vi "Log_Errors_20190313.vi"(7 "LoopName":string, 10 "error in":errorcluster) -> (2 "error out":errorcluster)   [LabVIEW 2021]
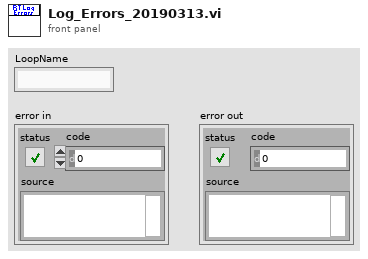
[diagram p1: front panel]
types:
  T1 = enum16{"open", "replace", "create", "open or create", "replace or create", "replace or create with confirmation"}
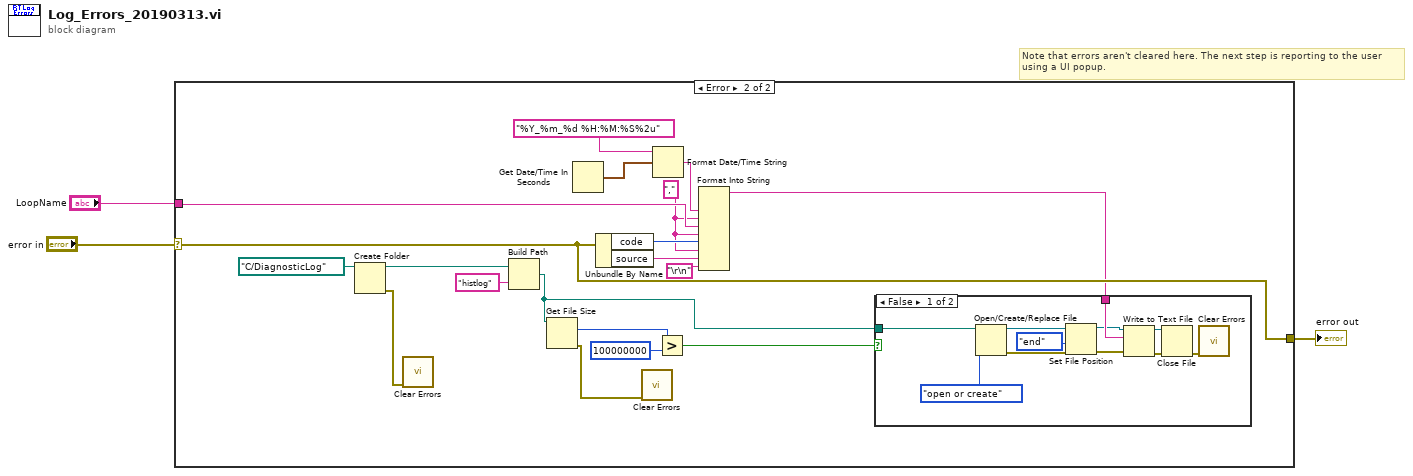
[diagram p0: block diagram]
diagram:
  # "Note that errors aren't cleared here. The next step is reporting to the user\nusing a UI popup."
  n1 = case shown="Error" "error in" {
    selector: "error in" -> [w4 w17]
    tunnel: [w4 w17] -> w2
    tunnel: "LoopName" -> [_ w23]
    frame No Error {
    }
    frame Error {
      w10 = "," ("source")
      n2 = Create Folder(path (use dialog)=path "C:/DiagnosticLog" ("file path (use dialog)")) -> (created path=w19:path, error out=w7:errorcluster)  [unwired: 2 in, 1 out]
      n3 = call <vilib>:"Clear Errors.vi"("error in (no error)"=w7) -> ()  [unwired: 5 in, 2 out]
      n4 = Build Path(base path=w19, name or relative path="histlog") -> (appended path=w5:path)
      n5 = Get File Size(file=w5) -> (size (in bytes)=w22:i64, 0:w8:errorcluster)  [unwired: 1 in, 1 out]
      n6 = Get Date/Time In Seconds() -> (seconds since 1Jan1904=w15:timestamp)
      n7 = Unbundle By Name(w17) -> ("code"=w11:i32, "source"=w12:string)
      n8 = call <vilib>:"Clear Errors.vi"("error in (no error)"=w8) -> ()  [unwired: 5 in, 2 out]
      n9 = Format Date/Time String(time format string (%c)="%Y_%m_%d %H:%M:%S%2u", seconds (now)=w15) -> (date/time string=w16:string)  [unwired: 1 out]
      n10 = Greater?(x=w22, y=i64 100000000) -> (0:w6:bool)
      n11 = Format Into String(w16, w10, w23, w10, w11, w10, w12, "\r\n") -> (resulting string=w14:string)  [unwired: 3 in, 1 out]
      n12 = case shown="False" w6 {
        tunnel: w14 -> [w34 _]
        tunnel: w5 -> [w24 _]
        frame False {
          n13 = Open/Create/Replace File(file path (use dialog)=w24, operation (0:open)=T1."open or create") -> (refnum out=w30:refnum<file>, error out=w27:errorcluster)  [unwired: 1 in, 4 out]
          n14 = Set File Position(refnum=w30, from (0:start)=enum16{"start", "end", "current"}."end", error in=w27) -> (refnum out=w31:refnum<file>, error out=w28:errorcluster)  [unwired: 1 out]
          n15 = Write to Text File(file (use dialog)=w31, text=w34, error in=w28) -> (refnum out=w32:refnum<file>, error out=w29:errorcluster)  [unwired: 2 out]
          n16 = Close File(refnum=w32, error in=w29) -> (error out=w25:errorcluster)  [unwired: 1 out]
          n17 = call <vilib>:"Clear Errors.vi"("error in (no error)"=w25) -> ()  [unwired: 5 in, 2 out]
        }
        frame True {
        }
      }
    }
  }
  "error out" <- w2
